vi "2_ImClass(Eval).vi"() -> ()   [LabVIEW 2020]
doc: "This example demonstrates the usage of Deep Learning Toolkit for solving hand written digit recognition problem with Convolutional Neural Network (CNN).\n\nDataset: MNIST http://yann.lecun.com/exdb/mnist/\nRequirements: Deep Learning Toolkit for LabVIEW."
uses:
  Controls/Img_RGB.ctl
  <vilib>/Ngene/Deep Learning Toolkit/Toolkit/NN_Network/Controls/NN_Device.ctl
  <vilib>/Ngene/Deep Learning Toolkit/Toolkit/NN_Network/Controls/NN_Save_Before_Destroy_Options.ctl
  <vilib>/Ngene/Deep Learning Toolkit/Toolkit/NN_Network/subVIs/NN_Predict/NN_Predict(In3D_Out1D).vi
  <vilib>/Ngene/Deep Learning Toolkit/Toolkit/NN_Train/Eval_Loss/NN_Eval_Test_Error_Loss/NN_Eval(In3D_Out1D).vi
  <vilib>/Ngene/Deep Learning Toolkit/Toolkit/NN_Train/Eval_Loss/NN_Calc_Cofusion_Matrix/NN_Calc_Confusion_Matrix(In3D_Out1D).vi
  <vilib>/Ngene/Deep Learning Toolkit/Toolkit/NN_Data/subVIs/Dataset_Destroy/NN_Dataset_Destroy(In3D_Out1D).vi
  <vilib>/Ngene/Deep Learning Toolkit/Toolkit/Deep_Learning_Toolkit_by_Ngene.lvlib
panel:
  out "Loss":dbl=0.46153685450553894
  out "Error Rate":dbl=0.15330000221729279
  out "Incorrectly Classified Imgs":T1[][](array[typedef])=[[{"image"=bytes[30030], "Truth"="airplane", "Predicted"="cat", "Name"="airplane_00077.bmp"}, {"image"=bytes[30030], "Truth"="airplane", "Predicted"="ship", "Name"="airplane_00093.bmp"}, {"image"=bytes[30030], "Truth"="airplane", "Predicted"="automobile", "Name"="airplane_00165.bmp"}, {"image"=bytes[30030], "Truth"="airplane", "Predicted"="deer", "Name"="airplane_00179.bmp"}, {"image"=bytes[30030], "Truth"="airplane", "Predicted"="ship", "Name"="airplane_00189.bmp"}, {"image"=bytes[30030], "Truth"="airplane", "Predicted"="ship", "Name"="airplane_00223.bmp"}], [{"image"=bytes[30030], "Truth"="airplane", "Predicted"="automobile", "Name"="airplane_00233.bmp"}, {"image"=bytes[30030], "Truth"="airplane", "Predicted"="ship", "Name"="airplane_00293.bmp"}, {"image"=bytes[30030], "Truth"="airplane", "Predicted"="automobile", "Name"="airplane_00352.bmp"}, {"image"=bytes[30030], "Truth"="airplane", "Predicted"="bird", "Name"="airplane_00497.bmp"}, {"image"=bytes[30030], "Truth"="airplane", "Predicted"="ship", "Name"="airplane_00604.bmp"}, {"image"=bytes[30030], "Truth"="airplane", "Predicted"="automobile", "Name"="airplane_00614.bmp"}], [{"image"=bytes[30030], "Truth"="airplane", "Predicted"="bird", "Name"="airplane_00748.bmp"}, {"image"=bytes[30030], "Truth"="airplane", "Predicted"="dog", "Name"="airplane_00799.bmp"}, {"image"=bytes[30030], "Truth"="airplane", "Predicted"="ship", "Name"="airplane_00812.bmp"}, {"image"=bytes[30030], "Truth"="airplane", "Predicted"="automobile", "Name"="airplane_00843.bmp"}, {"image"=bytes[30030], "Truth"="airplane", "Predicted"="ship", "Name"="airplane_00872.bmp"}, {"image"=bytes[30030], "Truth"="airplane", "Predicted"="bird", "Name"="airplane_00911.bmp"}], [{"image"=bytes[30030], "Truth"="airplane", "Predicted"="cat", "Name"="airplane_00989.bmp"}, {"image"=bytes[30030], "Truth"="airplane", "Predicted"="ship", "Name"="airplane_01039.bmp"}, {"image"=bytes[30030], "Truth"="airplane", "Predicted"="bird", "Name"="airplane_01188.bmp"}, {"image"=bytes[30030], "Truth"="airplane", "Predicted"="bird", "Name"="airplane_01234.bmp"}, {"image"=bytes[30030], "Truth"="airplane", "Predicted"="ship", "Name"="airplane_01382.bmp"}, {"image"=bytes[30030], "Truth"="airplane", "Predicted"="automobile", "Name"="airplane_01454.bmp"}], [{"image"=bytes[30030], "Truth"="airplane", "Predicted"="automobile", "Name"="airplane_01470.bmp"}, {"image"=bytes[30030], "Truth"="airplane", "Predicted"="bird", "Name"="airplane_01473.bmp"}, {"image"=bytes[30030], "Truth"="airplane", "Predicted"="horse", "Name"="airplane_01481.bmp"}, {"image"=bytes[30030], "Truth"="airplane", "Predicted"="truck", "Name"="airplane_01507.bmp"}, {"image"=bytes[30030], "Truth"="airplane", "Predicted"="bird", "Name"="airplane_01522.bmp"}, {"image"=bytes[30030], "Truth"="airplane", "Predicted"="automobile", "Name"="airplane_01560.bmp"}], [{"image"=bytes[30030], "Truth"="airplane", "Predicted"="ship", "Name"="airplane_01607.bmp"}, {"image"=bytes[30030], "Truth"="airplane", "Predicted"="truck", "Name"="airplane_01954.bmp"}, {"image"=bytes[30030], "Truth"="airplane", "Predicted"="automobile", "Name"="airplane_02010.bmp"}, {"image"=bytes[30030], "Truth"="airplane", "Predicted"="ship", "Name"="airplane_02021.bmp"}, {"image"=bytes[30030], "Truth"="airplane", "Predicted"="bird", "Name"="airplane_02233.bmp"}, {"image"=bytes[30030], "Truth"="airplane", "Predicted"="ship", "Name"="airplane_02248.bmp"}], [{"image"=bytes[30030], "Truth"="airplane", "Predicted"="automobile", "Name"="airplane_02413.bmp"}, {"image"=bytes[30030], "Truth"="airplane", "Predicted"="bird", "Name"="airplane_02421.bmp"}, {"image"=bytes[30030], "Truth"="airplane", "Predicted"="bird", "Name"="airplane_02429.bmp"}, {"image"=bytes[30030], "Truth"="airplane", "Predicted"="truck", "Name"="airplane_02622.bmp"}, {"image"=bytes[30030], "Truth"="airplane", "Predicted"="ship", "Name"="airplane_02659.bmp"}, {"image"=bytes[30030], "Truth"="airplane", "Predicted"="ship", "Name"="airplane_02675.bmp"}], [{"image"=bytes[30030], "Truth"="airplane", "Predicted"="bird", "Name"="airplane_02773.bmp"}, {"image"=bytes[30030], "Truth"="airplane", "Predicted"="ship", "Name"="airplane_02848.bmp"}, {"image"=bytes[30030], "Truth"="airplane", "Predicted"="ship", "Name"="airplane_02949.bmp"}, {"image"=bytes[30030], "Truth"="airplane", "Predicted"="ship", "Name"="airplane_02950.bmp"}, {"image"=bytes[30030], "Truth"="airplane", "Predicted"="ship", "Name"="airplane_03024.bmp"}, {"image"=bytes[30030], "Truth"="airplane", "Predicted"="automobile", "Name"="airplane_03204.bmp"}], [{"image"=bytes[30030], "Truth"="airplane", "Predicted"="automobile", "Name"="airplane_03337.bmp"}, {"image"=bytes[30030], "Truth"="airplane", "Predicted"="bird", "Name"="airplane_03438.bmp"}, {"image"=bytes[30030], "Truth"="airplane", "Predicted"="ship", "Name"="airplane_03441.bmp"}, {"image"=bytes[30030], "Truth"="airplane", "Predicted"="bird", "Name"="airplane_03549.bmp"}, {"image"=bytes[30030], "Truth"="airplane", "Predicted"="truck", "Name"="airplane_03570.bmp"}, {"image"=bytes[30030], "Truth"="airplane", "Predicted"="truck", "Name"="airplane_03647.bmp"}], [{"image"=bytes[30030], "Truth"="airplane", "Predicted"="truck", "Name"="airplane_03665.bmp"}, {"image"=bytes[30030], "Truth"="airplane", "Predicted"="ship", "Name"="airplane_03725.bmp"}, {"image"=bytes[30030], "Truth"="airplane", "Predicted"="automobile", "Name"="airplane_03880.bmp"}, {"image"=bytes[30030], "Truth"="airplane", "Predicted"="truck", "Name"="airplane_03938.bmp"}, {"image"=bytes[30030], "Truth"="airplane", "Predicted"="truck", "Name"="airplane_03964.bmp"}, {"image"=bytes[30030], "Truth"="airplane", "Predicted"="deer", "Name"="airplane_03987.bmp"}]]
  out "Confusion Matrix":string[][](table)=[["850", "4", "40", "7", "12", "1", "0", "13", "42", "31", "0.8500"], ["14", "919", "1", "1", "0", "0", "2", "2", "8", "53", "0.9190"], ["38", "1", "779", "24", "58", "29", "51", "11", "7", "2", "0.7790"], ["13", "3", "56", "658", "47", "132", "56", "20", "10", "5", "0.6580"], ["4", "3", "39", "19", "866", "10", "23", "34", "2", "0", "0.8660"], ["7", "2", "32", "101", "32", "778", "16", "26", "2", "4", "0.7780"], ["6", "3", "30", "23", "17", "12", "902", "2", "4", "1", "0.9020"], ["8", "0", "16", "24", "50", "24", "2", "870", "2", "4", "0.8700"], ["43", "13", "7", "4", "4", "3", "4", "1", "909", "12", "0.9090"], ["10", "26", "4", "8", "1", "1", "2", "4", "8", "936", "0.9360"], ["0.8560", "0.9435", "0.7759", "0.7572", "0.7967", "0.7859", "0.8526", "0.8850", "0.9145", "0.8931", ""]]
  in  "Dataset Path (Images)":path=path "D:/DNN/CIFAR-10_Images/Test"
  in  "NN_Device":T2=enum."GPU"
  in  "Weight File Path":path=path "D:/working/ImClass/ImClass_weights_25_04_18__18_42_33.bin"
  in  "Network Configuration File Path":path=path "D:/working/ImClass/ImClass_net_cfg_25_04_18__18_42_33.cfg"
  # "Overview:\nThis VI demonstrates how to evaluate performance of a trained model.\nRequirements: Deep Learning Toolkit for LabVIEW.\nInstructions:\n1. Set network topology .cfg file in the \"Network Configuration File Path\" control and trained weights .bin file in the \"Weight File Path\" control.\n2. Provide the test dataset path in the \"Dataset Path (Images)\" .\n3. Run the VI to evaluate the model's performance."
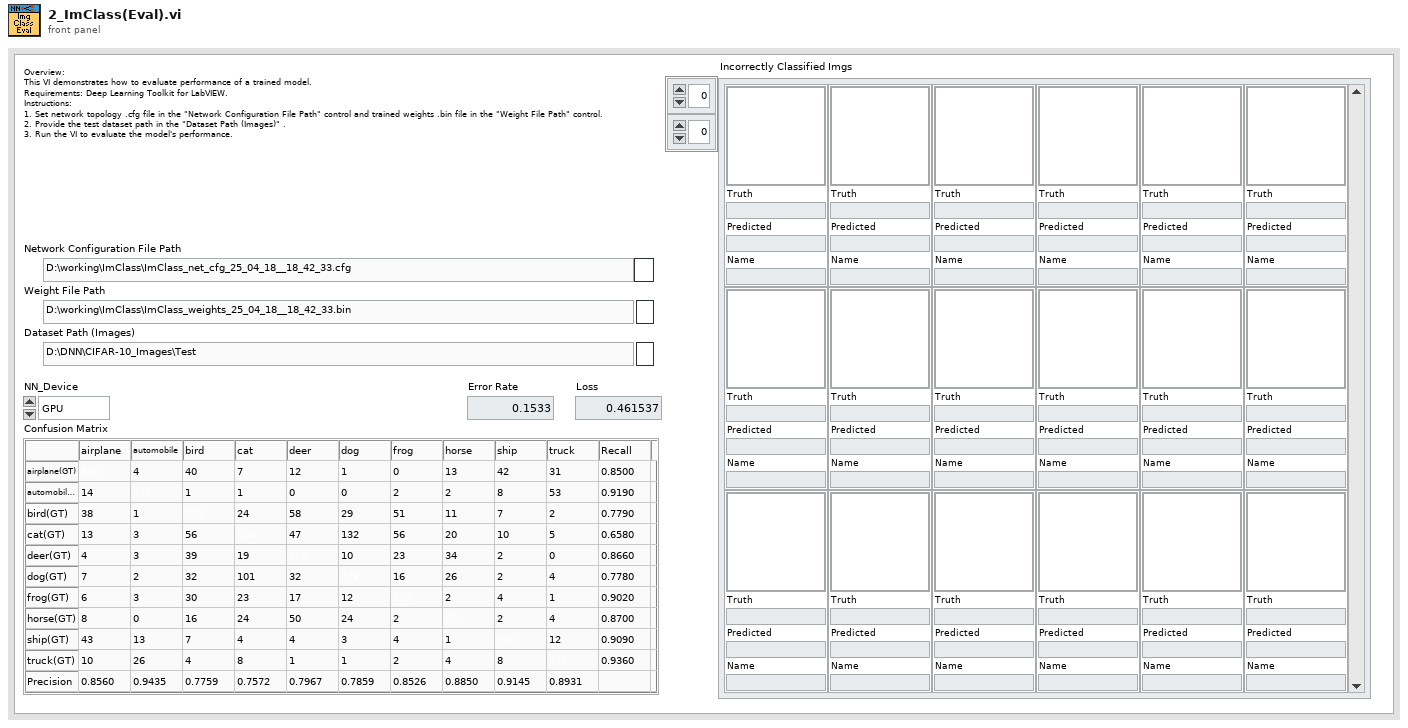
[diagram p1: front panel]
types:
  T1 = typedef "Img_RGB.ctl" = cluster{"image":picture, "Truth":string, "Predicted":string, "Name":string}
  T2 = typedef "Deep_Learning_Toolkit_by_Ngene.lvlib/NN_Device.ctl" = enum16{"CPU", "GPU"}
  T3 = typedef "Deep_Learning_Toolkit_by_Ngene.lvlib/NN_Save_Before_Destroy_Options.ctl" = cluster{"CFG?":bool, "Weights?":bool, "Render?":bool}
  T4 = typedef "Deep_Learning_Toolkit_by_Ngene.lvlib/NN_Config_Params.ctl" = cluster{"Name":string, "mBatch":i32, "NN_Train_Params":T5, "LR_Decay_Policy":T8, "Labels":string[], "Loss":T10}
  T5 = typedef "Deep_Learning_Toolkit_by_Ngene.lvlib/NN_Train_Params.ctl" = cluster{"Optimizer":T6, "Beta_1":sgl, "Beta_2":sgl, "Weight Decay(L1)":sgl, "Weight Decay(L2)":sgl, "Data_Sampling":T7}
  T6 = typedef "Deep_Learning_Toolkit_by_Ngene.lvlib/NN_Train_Optimizer.ctl" = enum16{"SGD", "Adam", "Adagrad", "Adadelta", "RMSProp", "Nesterov"}
  T7 = typedef "Deep_Learning_Toolkit_by_Ngene.lvlib/NN_Train_Data_Sampling.ctl" = enum16{"Random", "Sequential"}
  T8 = typedef "Deep_Learning_Toolkit_by_Ngene.lvlib/NN_LR_Policy_Cfg.ctl" = cluster{"Policy_Type":T9, "LR0":dbl, "k":sgl, "WarmUp_Policy":enum16{"Step", "Ramp"}, "WarmUp_Iter":i32, "WarmUp_Ratio":sgl}
  T9 = typedef "Deep_Learning_Toolkit_by_Ngene.lvlib/NN_LR_Policy_Type.ctl" = enum16{"Manual", "Step", "Exp", "1/t"}
  T10 = typedef "Deep_Learning_Toolkit_by_Ngene.lvlib/NN_Loss_Config_Params.ctl" = cluster{"Loss_Type":T11, "Loss_Conf_Params":variant}
  T11 = typedef "Deep_Learning_Toolkit_by_Ngene.lvlib/NN_Loss_Type.ctl" = enum16{"None", "MSE", "CrossEntropy", "YOLO_v2", "YOLO_v4"}
  T12 = typedef "Deep_Learning_Toolkit_by_Ngene.lvlib/NN_Layer_Config_Params.ctl" = cluster{"Layer_Type":T13, "Layer_Conf_Params":variant, "Input Layers":string[]}
  T13 = typedef "Deep_Learning_Toolkit_by_Ngene.lvlib/NN_Layer_Type.ctl" = enum16{"Input1D", "Input3D", "Conv1D", "Conv2D", "Conv2D_Adv", "MaxPool", "AvgPool", "UpSample", "DropOut3D", "ShortCut", "Concat", "SoftMax3D", "FC", "DropOut", "Softmax", "Flatten", "YOLO_v2", "YOLO_v4", "Activation", "BatchNormalization", "Unsupported"}
  T14 = typedef "Deep_Learning_Toolkit_by_Ngene.lvlib/NN.ctl" = cluster{"Name":string, "No of Layers":i32, "mBatch":i32, "Layers":T15[], "Dimty":T16, "Dims_In":T17, "Dims_Out":T17, "Working_Dir":path, "Train?":bool, "Train_Params":T5, "LR_Update_Policy":T8, "Session Data":T18, "Ground_truth":T19, "NNg_hdls":T20, "NN_Device":T2, "GPU Id":i32, "Labels":string[], "Receptive Field":T21[], "Loss_Type":T11, "Loss_Cfg_Prms":variant, "NNG_WS":T22}
  T15 = typedef "Deep_Learning_Toolkit_by_Ngene.lvlib/NN_Layer_ref.ctl" = refnum<data-value>
  T16 = typedef "Deep_Learning_Toolkit_by_Ngene.lvlib/NN_In_Out_Dim-ty.ctl" = enum8{"In1D_Out1D", "In3D_Out1D", "In3D_Out3D", "In3D_OutBBox"}
  T17 = typedef "Deep_Learning_Toolkit_by_Ngene.lvlib/NN_Dims(C,H,W).ctl" = cluster{"C":i32, "H":i32, "W":i32}
  T18 = typedef "Deep_Learning_Toolkit_by_Ngene.lvlib/NN_Train_Session_Data.ctl" = cluster{"Epochs":sgl, "Tot_Iter":i32, "LR":sgl, "LR_iter":i32}
  T19 = typedef "Deep_Learning_Toolkit_by_Ngene.lvlib/NN_Ground_truth.ctl" = cluster{"Y":variant}
  T20 = typedef "Deep_Learning_Toolkit_by_Ngene.lvlib/nng_cuda_handles.ctl" = cluster{"cudnn":u64, "cublas":u64, "stream":u64, "curand":u64}
  T21 = typedef "Deep_Learning_Toolkit_by_Ngene.lvlib/NN_Dims(V,H).ctl" = cluster{"V":i32, "H":i32}
  T22 = typedef "Deep_Learning_Toolkit_by_Ngene.lvlib/NNG_WS.ctl" = cluster{"NNG_WS_Mem":T23, "Max_WS_Size":i64}
  T23 = typedef "Deep_Learning_Toolkit_by_Ngene.lvlib/NNg_WS_Mem_DVR.ctl" = refnum<data-value>
  T24 = typedef "Deep_Learning_Toolkit_by_Ngene.lvlib/NN_DataSet(In3D_Out1D).ctl" = cluster{"Inputs Ref.":variant, "Outputs Ref.":T25, "Dataset_Size":i32, "Dims_In":T17, "Dims_Out":i32, "Labels":string[], "File Paths":path[]}
  T25 = typedef "Deep_Learning_Toolkit_by_Ngene.lvlib/NN_Data_ref(2D_SGL).ctl" = refnum<data-value>
  T26 = typedef "Deep_Learning_Toolkit_by_Ngene.lvlib/NN_Eval_Params.ctl" = cluster{"Loss":sgl, "Error":sgl}
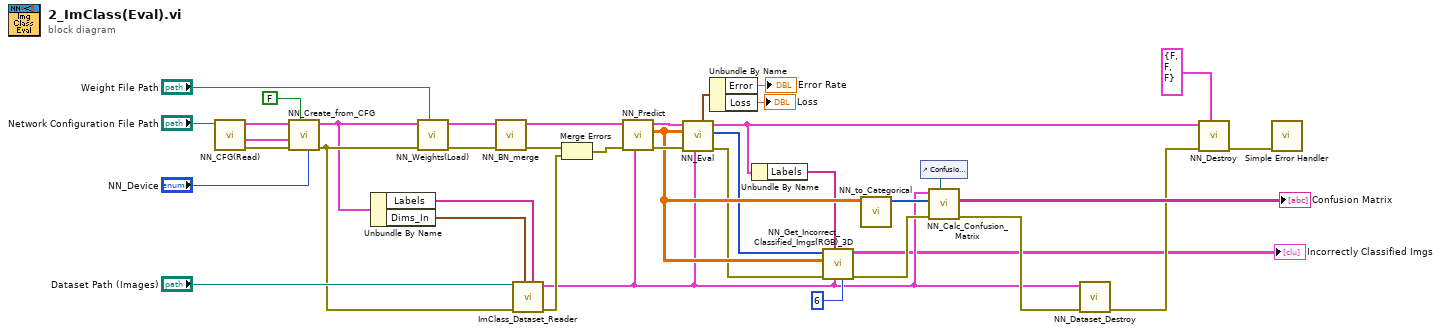
[diagram p0: block diagram]
diagram:
  n1 = call <vilib>:"NN_CFG(Read).vi"("CFG file path"="Network Configuration File Path") -> ("error out"=w20:errorcluster, "Net_Cfg"=w21:T4, "Layer_Cfg"=w19:T12[])  [unwired: 8 in]
  n2 = call <vilib>:"NN_Create_from_CFG.vi"("NN_Device"="NN_Device", "Train? (false)"=FALSE, "error in (no error)"=w20, "Net_Cfg"=w21, "Layer_Cfg"=w19) -> ("error out"=w10:errorcluster, "NN out"=w3:T14)  [unwired: 5 in]
  n3 = Unbundle By Name(w3) -> ("Labels"=w2:string[], "Dims_In"=w1:T17)
  n4 = call <vilib>:"NN_Weights(Load).vi"("Weight File Path"="Weight File Path", "error in (no error)"=w10, "NN in"=w3) -> ("error out"=w15:errorcluster, "NN out"=w16:T14)  [unwired: 7 in]
  n5 = call <vilib>:"NN_BN_merge.vi"("error in (no error)"=w15, "NN in"=w16) -> ("error out"=w13:errorcluster, "NN out"=w14:T14)  [unwired: 8 in]
  n6 = call "ImClass_Dataset_Reader.vi"("Unique labels"=w2, "Dims(C,H,W)"=w1, "error in (no error)"=w10, "Image Foldr Path"="Dataset Path (Images)") -> ("error out"=w8:errorcluster, "NN_DataSet(In3D_OutBBox)"=w5:T24)  [unwired: 6 in]
  n7 = Merge Errors(w13, w8) -> (w9:errorcluster)
  n8 = call-poly <vilib>:"NN_Predict.vi"("Dataset"=w5, "error in (no error)"=w9, "NN in"=w14) -> ("error out"=w34:errorcluster, "Predictions"=w32:sgl[][], "NN out"=w35:T14)  [unwired: 6 in]
  n9 = call-poly <vilib>:"NN_Eval.vi"("Dataset"=w5, "error in (no error)"=w34, "Predictions"=w32, "NN in"=w35) -> ("error out"=w31:errorcluster, "Incrct_Class_idx"=w29:i32[], "NN out"=w25:T14, "NN_Eval_Params"=w26:T26)  [unwired: 4 in]
  n10 = Unbundle By Name(w26) -> ("Error"=→"Error Rate":sgl, "Loss"=→"Loss":sgl)
  n11 = Unbundle By Name(w25) -> ("Labels"=w24:string[])
  n12 = call "NN_Get_Incorrect_Classified_Imgs(RGB)_3D.vi"("# of columns"=6 ("Report shape"), "Dataset"=w5, "Labels"=w24, "error in (no error)"=w31, "Predictions"=w32, "MisClassed_idx"=w29) -> ("error out"=w30:errorcluster, "Images(GrayScale)"=→"Incorrectly Classified Imgs":T1[][])  [unwired: 4 in]
  n13 = call <vilib>:"NN_to_Categorical.vi"("Prediction"=w32) -> ("Label_Idx"=w33:i32[])  [unwired: 10 in]
  n14 = control-ref of="Confusion Matrix"() -> (w36:refnum<vi>)
  n15 = call-poly <vilib>:"NN_Calc_Confusion_Matrix.vi"("Confusion Matrix (Table) ref."=w36, "error in (no error)"=w30, "Predictions"=w33, "Dataset"=w5) -> ("error out"=w7:errorcluster, "Confusion Matrix (Table)"=→"Confusion Matrix":string[][])  [unwired: 3 in, 3 out]
  n16 = call-poly <vilib>:"NN_Dataset_Destroy.vi"("error in (no error)"=w7, "Dataset(In3D_Out1D)"=w5) -> ("error out"=w6:errorcluster)  [unwired: 9 in]
  n17 = call <vilib>:"NN_Destroy.vi"("Save (T, T, T)"=T3 {"CFG?"=FALSE, "Weights?"=FALSE, "Render?"=FALSE} ("Save_Config"), "error in (no error)"=w6, "NN in"=w25) -> ("error out"=w39:errorcluster)  [unwired: 7 in, 1 out]
  n18 = call <vilib>:"Simple Error Handler.vi"("error in (no error)"=w39) -> ()  [unwired: 4 in, 5 out]
